vi "FW_create_folder.vi"(7 "Decimate_frameRate":i32=1, 8 "error in (no error)":errorcluster, 9 "frame_offset":i32=1, 10 "amount_frames":u32=1, 11 "Path":path) -> (0 "error out":errorcluster, 3 "created path":path)   [LabVIEW 2021, in "Framework_lib.lvlib"]
uses:
  QMH/Framework_lib.lvlib
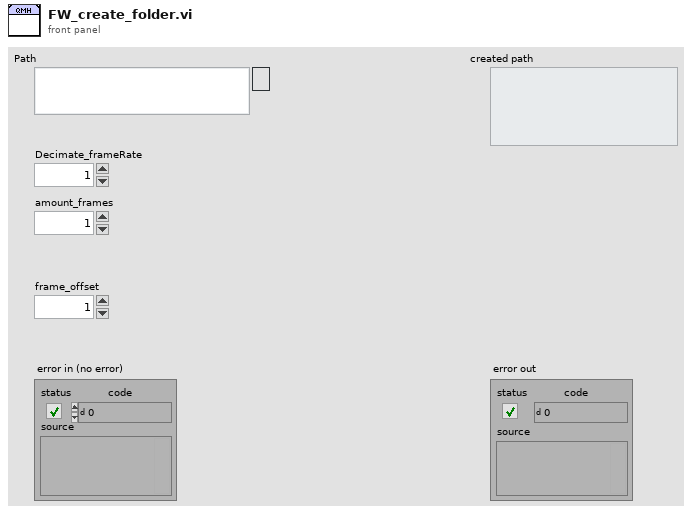
[diagram p1: front panel]
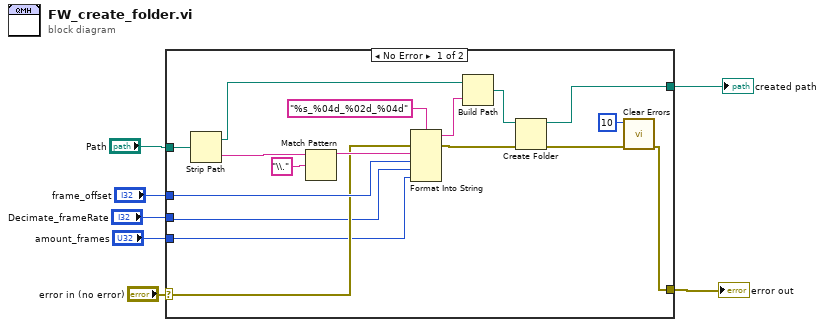
[diagram p0: block diagram]
diagram:
  n1 = case shown="No Error" "error in (no error)" {
    selector: "error in (no error)" -> [w15 w25]
    tunnel: "amount_frames" -> [w8 _]
    tunnel: "frame_offset" -> [w21 _]
    tunnel: "Path" -> [w16 _]
    tunnel: [w12 _] -> w3
    tunnel: [w11 w25] -> w2
    tunnel: "Decimate_frameRate" -> [w9 _]
    frame No Error {
      n2 = Strip Path(path=w16) -> (stripped path=w22:path, name=w18:string)
      n3 = Match Pattern(string=w18, regular expression="\\.") -> (before substring=w20:string)  [unwired: 1 in, 3 out]
      n4 = Format Into String(format string="%s_%04d_%02d_%04d", error in=w15, w20, w21, w9, w8) -> (resulting string=w23:string, error out=w14:errorcluster)  [unwired: 1 in]
      n5 = Build Path(base path=w22, name or relative path=w23) -> (appended path=w24:path)
      n6 = Create Folder(path (use dialog)=w24, error in=w14) -> (created path=w12:path, error out=w13:errorcluster)  [unwired: 1 in, 1 out]
      n7 = call <vilib>:"Clear Errors.vi"("error in (no error)"=w13, "specific error code to clear (0: all)"=10) -> ("error out"=w11:errorcluster)  [unwired: 4 in, 1 out]
    }
    frame Error {
    }
  }
  "error out" <- w2
  "created path" <- w3
